vi "Generate Pretty Icon Text Layer.vi"(0 "Icon in":refnum<class "Icon.lvclass">, 5 "VI Name":string, 7 "Library Path":path, 9 "Number of Rows in Icon":i32, 11 "error in (no error)":errorcluster, 12 "Icon Height":i16) -> (4 "Icon out":refnum<class "Icon.lvclass">, 15 "error out":errorcluster)   [LabVIEW 2024, in "Text-Based VI Icon.lvlib"]
doc: "Generating the LV Icon Text Layer requires the Text cluster.\nIn addition to the Text, it is possible to specify the visual appearance of the Text as well as a default Template Layer glyph.\n\nThe default value for the visual appearance is:\nFont: Small Fonts\nAlignment: Center\nSize: 8\nCenter text vertically: TRUE\nCapitalize text: TRUE\nColor of all four lines: Black\n\nThe default value of the Template layer is:\nSize: 32 x 32\nBorder Color: Black\nBackground Color: White"
uses:
  <vilib>/LabVIEW Icon API/Set Text Icon/Text-Based VI Icon.lvlib
  <vilib>/LabVIEW Icon API/lv_icon/Classes/Icon/Icon.lvclass
  <vilib>/LabVIEW Icon API/API_Test Settings.ctl
  <vilib>/LabVIEW Icon API/lv_icon/Controls/Alignment.ctl
  <vilib>/LabVIEW Icon API/API_Text Colors.ctl
  <vilib>/LabVIEW Icon API/lv_icon/Controls/Graphic.ctl
  <vilib>/LabVIEW Icon API/lv_icon/Classes/Icon Framework/Icon Framework.lvclass
  <vilib>/LabVIEW Icon API/LabVIEW Icon API.lvlib
panel:
  in  "LayerName":string="Icon Text"
  # "`"
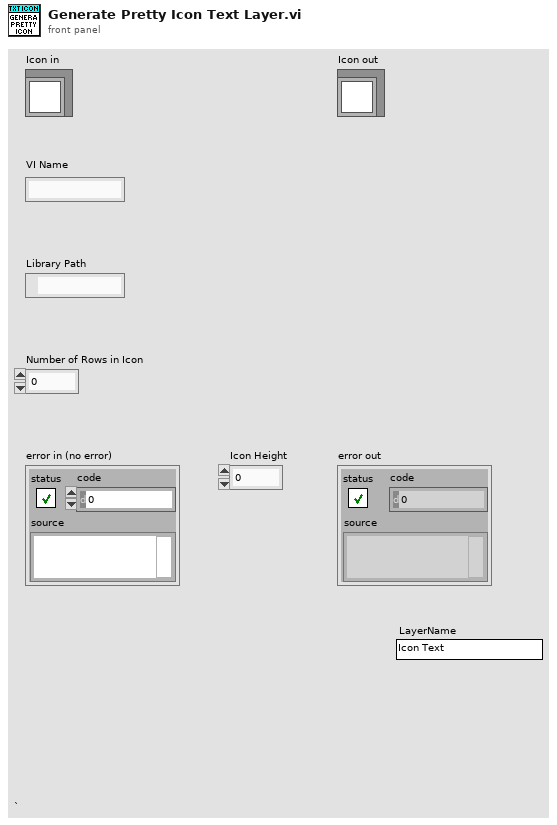
[diagram p1: front panel]
types:
  T1 = typedef "Graphic.ctl" = cluster{"Rectangle":cluster{"left":i16, "top":i16, "right":i16, "bottom":i16}, "Path":path, "Image":picture, "Filter":string, "FileName":string}
  T2 = typedef "LabVIEW Icon API.lvlib/API_Test Settings.ctl" = cluster{"Font":string, "Alignment":T3, "Size":u8, "Center text":bool, "Capitalize text":bool, "Text color":T4}
  T3 = typedef "Alignment.ctl" = u16
  T4 = typedef "LabVIEW Icon API.lvlib/API_Text Colors.ctl" = cluster{"Line 1 color":u32, "Line 2 color":u32, "Line 3 color":u32, "Line 4 color":u32}
  T5 = typedef "LabVIEW Icon API.lvlib/API_Text.ctl" = cluster{"Line 1 text":string, "Line 2 text":string, "Line 3 text":string, "Line 4 text":string}
  T6 = typedef "BodyText.ctl" = cluster{"Line 1 text":string, "Line 2 text":string, "Line 3 text":string, "Line 4 text":string, "Line 1 color":u32, "Line 2 color":u32, "Line 3 color":u32, "Line 4 color":u32, "Body Text Spec":cluster{"Font":T7, "Alignment":T3, "Size":u8}, "Center text vertically":bool, "Capitalize Text":bool}
  T7 = typedef "Font.ctl" = string
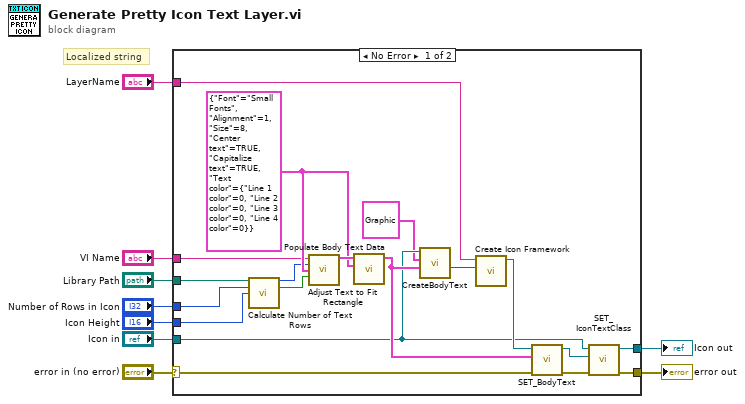
[diagram p0: block diagram]
diagram:
  # "Localized string"
  n1 = case shown="No Error" "error in (no error)" {
    selector: "error in (no error)" -> [w15 w30]
    tunnel: [w28 w30] -> w8
    tunnel: [w27 w29] -> w6
    tunnel: "Icon in" -> [w22 w29]
    tunnel: "VI Name" -> [w18 _]
    tunnel: "LayerName" -> [w16 _]
    tunnel: "Library Path" -> [w14 _]
    tunnel: "Number of Rows in Icon" -> [w13 _]
    tunnel: "Icon Height" -> [w11 _]
    frame No Error {
      w20 = T2 {"Font"="Small Fonts", "Alignment"=1, "Size"=8, "Center text"=TRUE, "Capitalize text"=TRUE, "Text color"={"Line 1 color"=0, "Line 2 color"=0, "Line 3 color"=0, "Line 4 color"=0}} ("Text settings")
      n2 = call <vilib>:"Calculate Number of Text Rows.vi"("Library Path"=w14, "Number of Pixel Rows in Icon"=w13, "Icon Height"=w11) -> ("Number of Text Rows"=w12:i32, "Blank Line 1 Text"=w10:bool)  [unwired: 11 in]
      n3 = call <vilib>:"Adjust Text to Fit Rectangle.vi"("VI Name"=w18, "Number of Rows"=w12, "Text settings"=w20, "Blank Line 1 text?"=w10) -> ("Text out"=w21:T5)  [unwired: 11 in]
      n4 = call <vilib>:"Populate Body Text Data.vi"("Text settings"=w20, "Text"=w21) -> ("Body Text"=w24:T6)  [unwired: 9 in]
      n5 = call <vilib>:"CreateBodyText.vi"("Body Text"=w24, "Path and Icon Template"=T1 {"Rectangle"={"left"=0, "top"=0, "right"=0, "bottom"=0}, "Path"=path "", "Image"=bytes[0], "Filter"="", "FileName"=""}, "Icon.lvclass in"=w22) -> ("Body Text"=w26:picture)  [unwired: 8 in]
      n6 = call <vilib>:"Create Icon Framework.vi"("Template Glyph"=w26, "Layer name"=w16) -> ("Icon Framework out"=w25:refnum<class "Icon Framework.lvclass">)  [unwired: 9 in]
      n7 = call-dynamic "SET_BodyText.vi"("error in (no error)"=w15, "Body Text"=w24, "Icon Framework.lvclass in"=w25) -> ("error out"=w17:errorcluster, "Icon Framework.lvclass out"=w23:refnum<class "Icon Framework.lvclass">)  [unwired: 7 in]
      n8 = call-dynamic "SET_IconTextClass.vi"("error in (no error)"=w17, "Icon Framework.lvclass"=w23, "Icon.lvclass in"=w22) -> ("error out"=w28:errorcluster, "Icon.lvclass out"=w27:refnum<class "Icon.lvclass">)  [unwired: 7 in]
    }
    frame Error {
    }
  }
  "error out" <- w8
  "Icon out" <- w6
